vi "aaa3.vi"() -> ()   [LabVIEW 2010]
uses:
  pair.ctl
panel:
  out "Array":T1[](array[typedef])
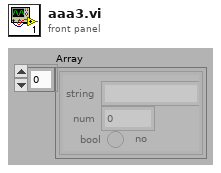
[diagram p1: front panel]
types:
  T1 = typedef "pair.ctl" = cluster{"num":i32, "bool":bool, "string":string}
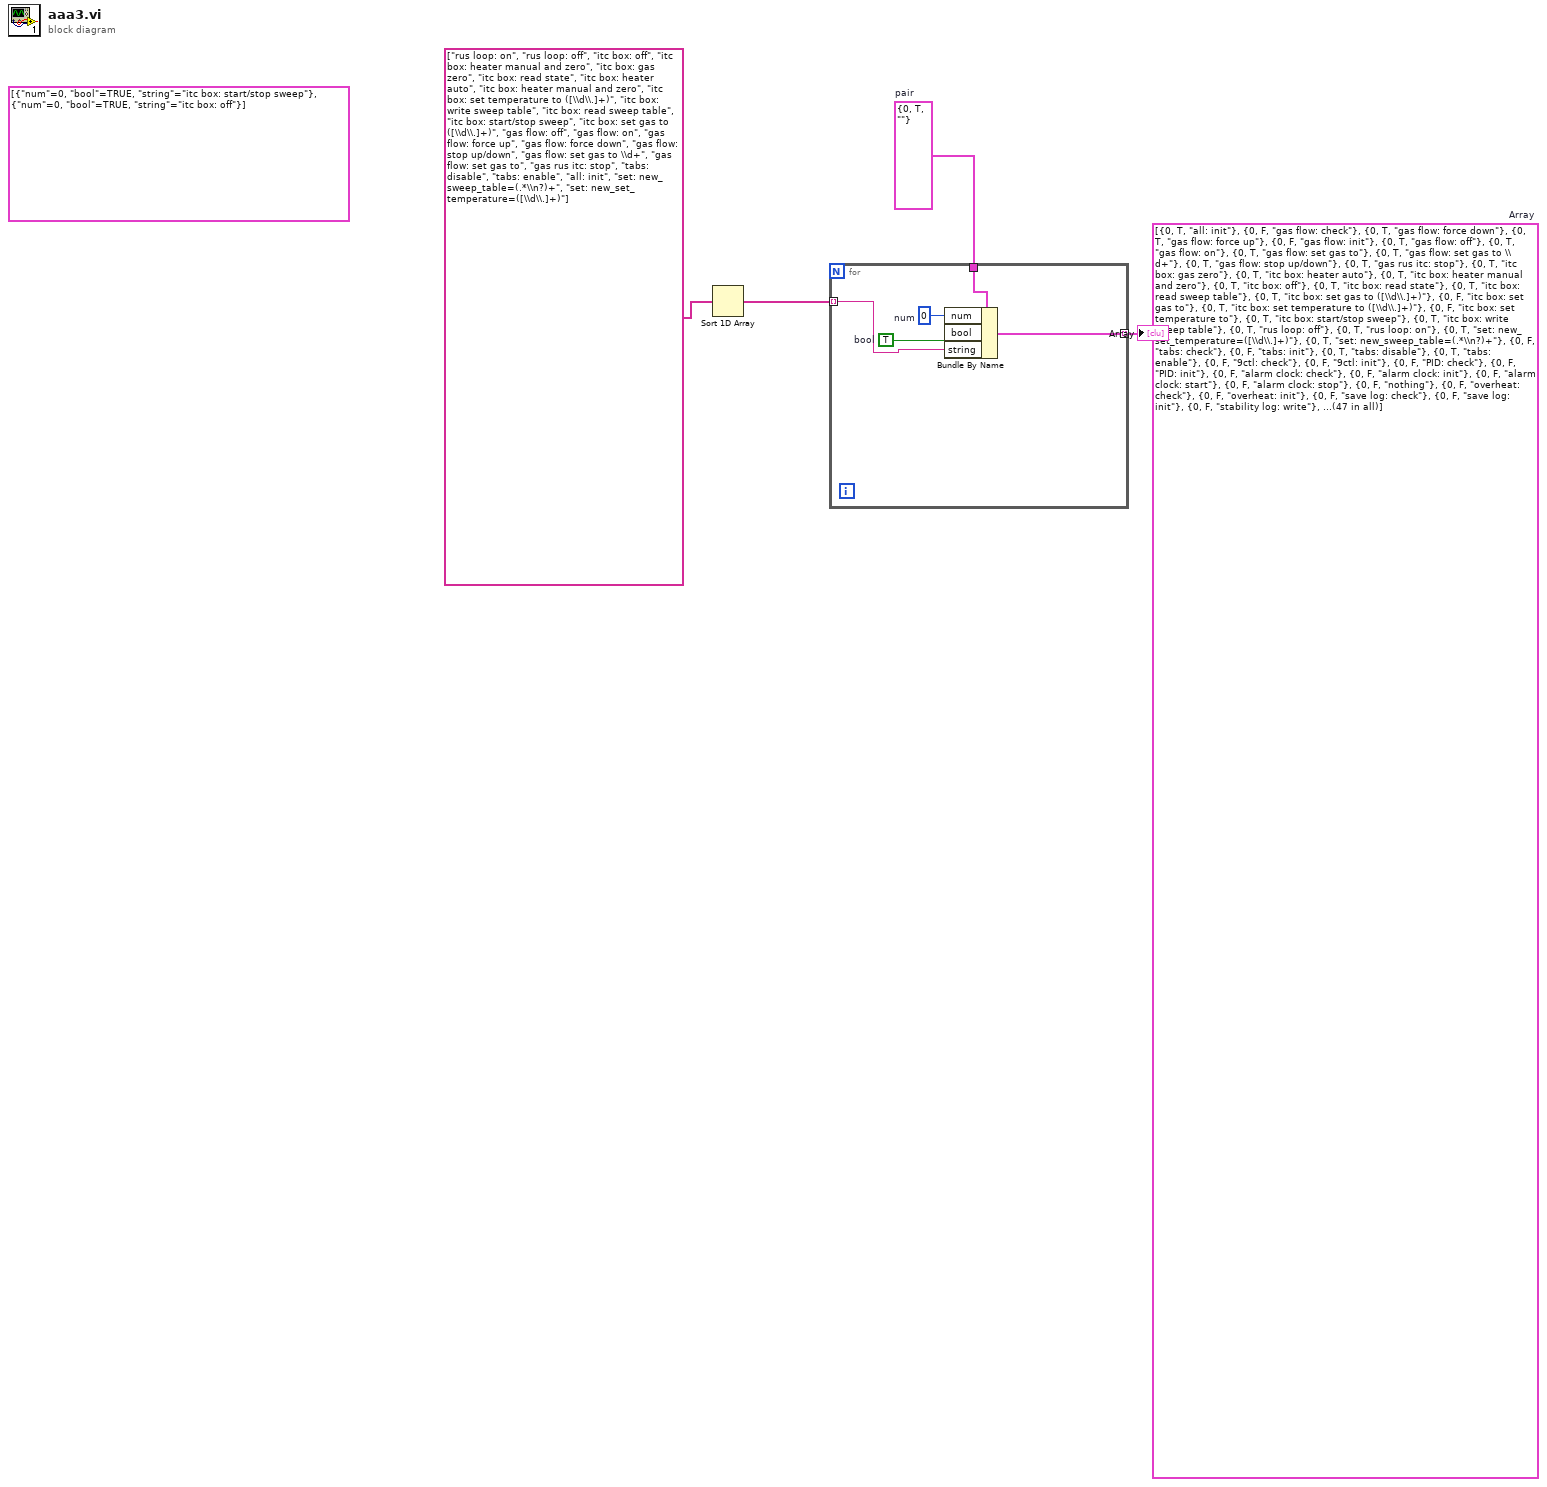
[diagram p0: block diagram]
diagram:
  (unwired) T1[] [{"num"=0, "bool"=TRUE, "string"="all: init"}, {"num"=0, "bool"=FALSE, "string"="gas flow: check"}, {"num"=0, "bool"=TRUE, "string"="gas flow: force down"}, {"num"=0, "bool"=TRUE, "string"="gas flow: force up"}, {"num"=0, "bool"=FALSE, "string"="gas flow: init"}, {"num"=0, "bool"=TRUE, "string"="gas flow: off"}, {"num"=0, "bool"=TRUE, "string"="gas flow: on"}, {"num"=0, "bool"=TRUE, "string"="gas flow: set gas to"}, {"num"=0, "bool"=TRUE, "string"="gas flow: set gas to \\d+"}, {"num"=0, "bool"=TRUE, "string"="gas flow: stop up/down"}, {"num"=0, "bool"=TRUE, "string"="gas rus itc: stop"}, {"num"=0, "bool"=TRUE, "string"="itc box: gas zero"}, {"num"=0, "bool"=TRUE, "string"="itc box: heater auto"}, {"num"=0, "bool"=TRUE, "string"="itc box: heater manual and zero"}, {"num"=0, "bool"=TRUE, "string"="itc box: off"}, {"num"=0, "bool"=TRUE, "string"="itc box: read state"}, {"num"=0, "bool"=TRUE, "string"="itc box: read sweep table"}, {"num"=0, "bool"=TRUE, "string"="itc box: set gas to ([\\d\\.]+)"}, {"num"=0, "bool"=FALSE, "string"="itc box: set gas to"}, {"num"=0, "bool"=TRUE, "string"="itc box: set temperature to ([\\d\\.]+)"}, {"num"=0, "bool"=FALSE, "string"="itc box: set temperature to"}, {"num"=0, "bool"=TRUE, "string"="itc box: start/stop sweep"}, {"num"=0, "bool"=TRUE, "string"="itc box: write sweep table"}, {"num"=0, "bool"=TRUE, "string"="rus loop: off"}, {"num"=0, "bool"=TRUE, "string"="rus loop: on"}, {"num"=0, "bool"=TRUE, "string"="set: new_set_temperature=([\\d\\.]+)"}, {"num"=0, "bool"=TRUE, "string"="set: new_sweep_table=(.*\\n?)+"}, {"num"=0, "bool"=FALSE, "string"="tabs: check"}, {"num"=0, "bool"=FALSE, "string"="tabs: init"}, {"num"=0, "bool"=TRUE, "string"="tabs: disable"}, {"num"=0, "bool"=TRUE, "string"="tabs: enable"}, {"num"=0, "bool"=FALSE, "string"="9ctl: check"}, {"num"=0, "bool"=FALSE, "string"="9ctl: init"}, {"num"=0, "bool"=FALSE, "string"="PID: check"}, {"num"=0, "bool"=FALSE, "string"="PID: init"}, {"num"=0, "bool"=FALSE, "string"="alarm clock: check"}, {"num"=0, "bool"=FALSE, "string"="alarm clock: init"}, {"num"=0, "bool"=FALSE, "string"="alarm clock: start"}, {"num"=0, "bool"=FALSE, "string"="alarm clock: stop"}, {"num"=0, "bool"=FALSE, "string"="nothing"}, {"num"=0, "bool"=FALSE, "string"="overheat: check"}, {"num"=0, "bool"=FALSE, "string"="overheat: init"}, {"num"=0, "bool"=FALSE, "string"="save log: check"}, {"num"=0, "bool"=FALSE, "string"="save log: init"}, {"num"=0, "bool"=FALSE, "string"="stability log: write"}, {"num"=0, "bool"=FALSE, "string"="sweep table: init"}, {"num"=0, "bool"=FALSE, "string"="sweep table: check"}]  # Array
  w2 = T1 {"num"=0, "bool"=TRUE, "string"=""}  # pair
  (unwired) T1[] [{"num"=0, "bool"=TRUE, "string"="itc box: start/stop sweep"}, {"num"=0, "bool"=TRUE, "string"="itc box: off"}]
  n1 = Sort 1D Array(array=string[] ["rus loop: on", "rus loop: off", "itc box: off", "itc box: heater manual and zero", "itc box: gas zero", "itc box: read state", "itc box: heater auto", "itc box: heater manual and zero", "itc box: set temperature to ([\\d\\.]+)", "itc box: write sweep table", "itc box: read sweep table", "itc box: start/stop sweep", "itc box: set gas to ([\\d\\.]+)", "gas flow: off", "gas flow: on", "gas flow: force up", "gas flow: force down", "gas flow: stop up/down", "gas flow: set gas to \\d+", "gas flow: set gas to", "gas rus itc: stop", "tabs: disable", "tabs: enable", "all: init", "set: new_sweep_table=(.*\\n?)+", "set: new_set_temperature=([\\d\\.]+)"]) -> (sorted array=w3:string[])
  n2 = for {
    tunnel: w3 -> [w6] mode=indexing
    tunnel: w2 -> [w9]
    tunnel: [w5] -> w1 mode=indexing
    w7 = TRUE  # bool
    w8 = 0  # num
    n3 = Bundle By Name(cluster=w9, "num"=w8, "bool"=w7, "string"=w6) -> (w5:T1)
  }
  "Array" <- w1
